vi "CloseCamera.vi"(3 "error in":errorcluster, 4 "Updated camera":T2, 5 "Saving":bool) -> (0 "error out":errorcluster, 2 "Saving out":bool)   [LabVIEW 2017]
doc: "Creates, and edits acquisitions using the NI Vision Acquisition Express VI.\n\nThe NI Vision Acquisition Wizard is launched by placing the Express VI on the block diagram. Select an acquisition source and configure an acquisition using NI-IMAQ, NI-IMAQdx, or simulate an acquisition by reading an AVI or image files from a folder. After an acquisition is configured, select controls and indicators to be able to programmatically set in LabVIEW. Double-click the Vision Acquisition Express VI to edit the acquisition.\n\nNote: Any images created by the Express VI need to be disposed after use. Use the IMAQ Dispose.vi to cleanup the images output by the Express VI when they are no longer needed."
uses:
  <vilib>/vision/Image Controls.llb/IMAQ Image.ctl
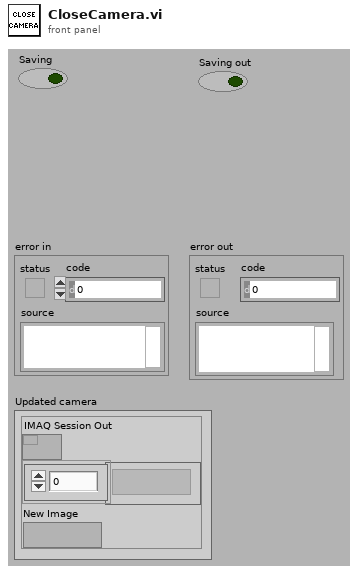
[diagram p1: front panel]
types:
  T1 = typedef "IMAQ Image.ctl" = refnum<image>
  T2 = cluster{"IMAQ Session Out":refnum<k11>, "Array":T1[], "New Image":T1}
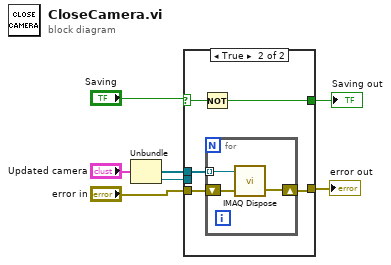
[diagram p0: block diagram]
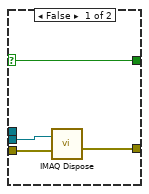
[diagram p2: hidden frame]
diagram:
  n1 = Unbundle("Updated camera") -> ("Array"=w1:T1[], "New Image"=w3:T1)  [unwired: 1 out]
  n2 = case shown="True" "Saving" {
    selector: "Saving" -> [w11 w16]
    tunnel: [w11 w15] -> w5
    tunnel: "error in" -> [w8 w13]
    tunnel: w3 -> [w10 _]
    tunnel: [w9 w12] -> w2
    tunnel: w1 -> [_ w14]
    frame False {
      n3 = call "IMAQ Dispose"("Image"=w10, "error in (no error)"=w8) -> ("error out"=w9:errorcluster)  [unwired: 4 in]
    }
    frame True {
      n4 = Not(x=w16) -> (.not. x?=w15:bool)
      n5 = for {
        tunnel: w14 -> [w19] mode=indexing
        shift-right: [w17] -> w12
        shift-left: w13 -> [w18]
        n6 = call "IMAQ Dispose"("Image"=w19, "error in (no error)"=w18) -> ("error out"=w17:errorcluster)  [unwired: 4 in]
      }
    }
  }
  "error out" <- w2
  "Saving out" <- w5
